vi "OpenExplorer.vi"() -> ()   [LabVIEW 2014]
panel:
  out "Folder path Out":path
  # "Display Folder in Windows Explorer programmatically"
  # "This vi will display a folder path in windows explorer by using system executive"
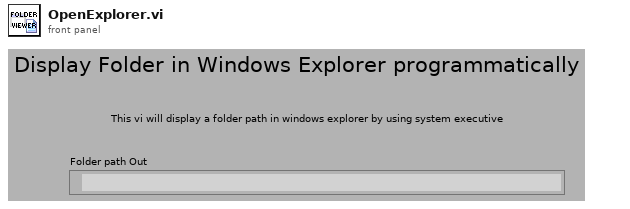
[diagram p1: front panel]
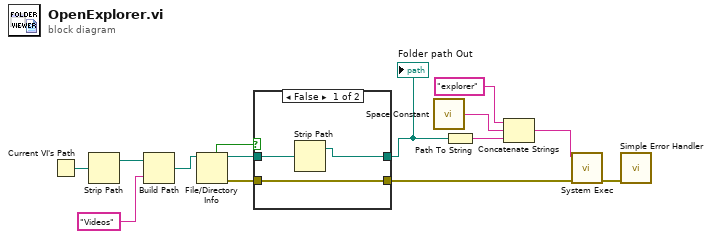
[diagram p0: block diagram]
diagram:
  n1 = Current VI's Path() -> (path=w4:path)
  n2 = Strip Path(path=w4) -> (stripped path=w3:path)  [unwired: 1 out]
  n3 = Build Path(base path=w3, name or relative path="Videos") -> (appended path=w1:path)
  n4 = File/Directory Info(path=w1) -> (path out=w11:path, directory=w7:bool, error out=w9:errorcluster)  [unwired: 1 in, 4 out]
  n5 = case shown="False" w7 {
    tunnel: w11 -> [w17 w19]
    tunnel: [w15 w19] -> w10
    tunnel: w9 -> [w16 w18]
    tunnel: [w16 w18] -> w8
    frame False {
      n6 = Strip Path(path=w17) -> (stripped path=w15:path)  [unwired: 1 out]
    }
    frame True {
    }
  }
  "Folder path Out" <- w10
  n7 = call <vilib>:"Space Constant.vi"() -> ("String"=w5:string)
  n8 = Path To String(path=w10) -> (string=w13:string)
  n9 = Concatenate Strings("explorer" ("string"), w5, w13) -> (w12:string)
  n10 = call <vilib>:"System Exec.vi"("error in (no error)"=w8, "command line"=w12) -> ("error out"=w14:errorcluster)  [unwired: 6 in, 3 out]
  n11 = call <vilib>:"Simple Error Handler.vi"("error in (no error)"=w14) -> ()  [unwired: 4 in, 5 out]
